vi "main_test3.vi"() -> ()   [LabVIEW 2018]
uses:
  <vilib>/addons/database/Connection.llb/DB Tools Open Connec (Path).vi
  <vilib>/addons/database/NI_Database_API.lvlib
panel:
  in  "确定按钮":bool
  out "数值":dbl format="%#.2g"
  in  "uid":i16
  in  "经度":sgl
  in  "纬度":sgl
  in  "温度":sgl=3.9
  out "时间":timestamp format="%<%H:%M:%S\n%Y/%m/%d>T"
  out "数据采集":bool=TRUE
  out "flaginit":bool=TRUE
  out "温度报警":string[][](table)
  out "疫苗信息":string[][](table)
  out "uid":i16
  out "途径地点":i32
  out "运输路径":cluster{"city":string, "布尔":T1}[](array[cluster])
  out "error out":errorcluster
  out "负责人信息":T2
  in  "CYJ":bool
  out "定位":bool
  out "温度":cluster{"元素":sgl, "温度":sgl, "元素":sgl}(graph)
  out "纬度":string
  out "经度":string
  in  "地图比例":i8(slide)=10 scale=6.0..18.0
  in  "地图":refnum<k7>(container) caption="网页浏览器"
  in  "Setvi":bool
  in  "停止":bool
  # "疫苗冷链储运监控系统\nVACCINE COLD-CHAIN TRANSPORTATION MONITORING SYSTEM"
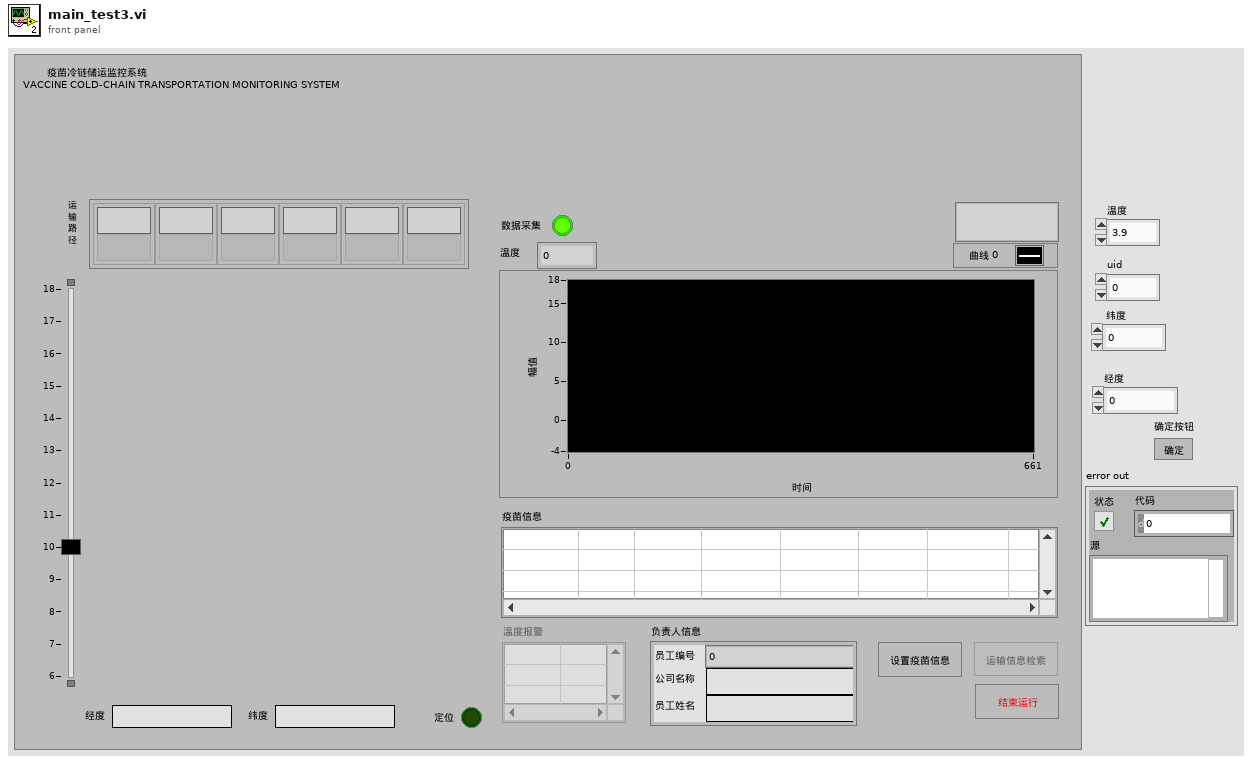
[diagram p1: front panel]
types:
  T1 = typedef "car.ctl" = bool
  T2 = typedef "人员信息.ctl" = cluster{"员工编号":i32, "公司名称":string, "员工姓名":string}
  T3 = typedef "储运信息.ctl" = cluster{"纬度":sgl, "经度":sgl, "温度":sgl, "负责人":i32, "区域":string, "记录时间":timestamp}
  T4 = enum8{"Enabled", "Disabled", "Disabled and Grayed Out"}
  T5 = typedef "NI_Database_API.lvlib/Conn ObjectReference.ctl" = refnum<k1>
  T6 = typedef "疫苗信息.ctl" = cluster{"疫苗名":string, "疫苗编号":i32, "疫苗类型":string, "生产厂家":string, "生产日期":timestamp, "生产地":string, "生产负责人":string, "是否合格":string, "疫苗功能":string}
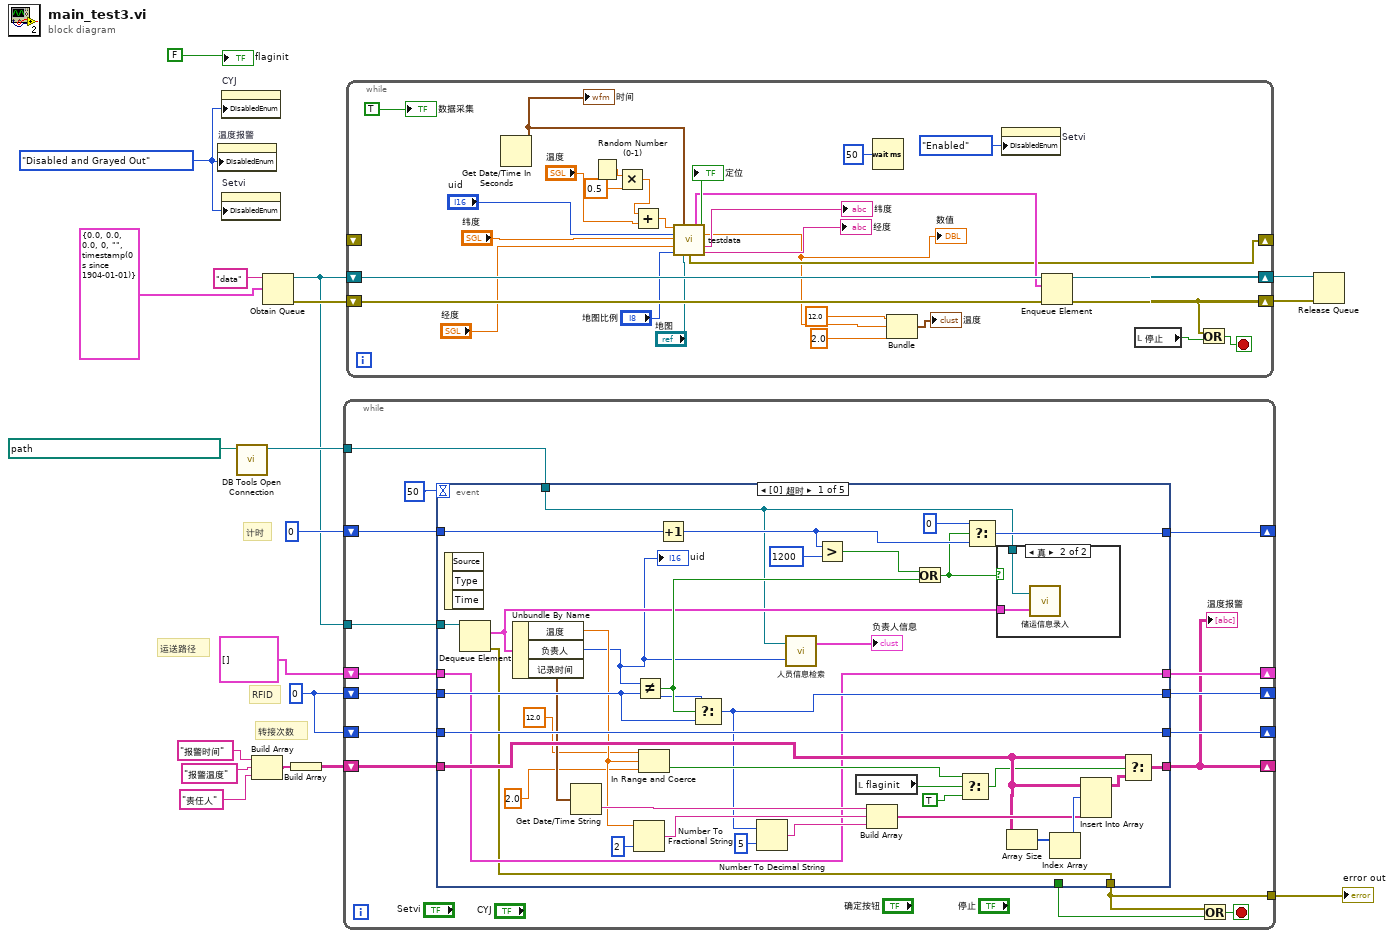
[diagram p0: block diagram]
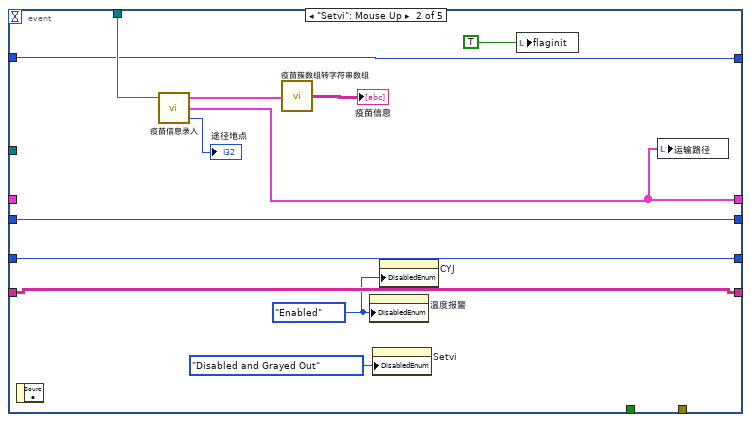
[diagram p3: hidden frame]
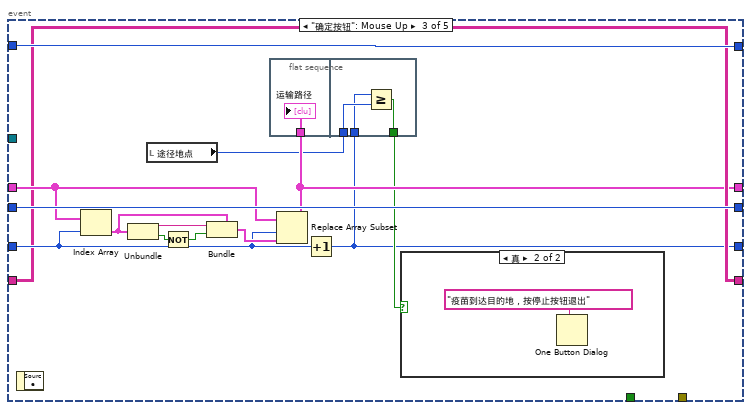
[diagram p4: hidden frame]
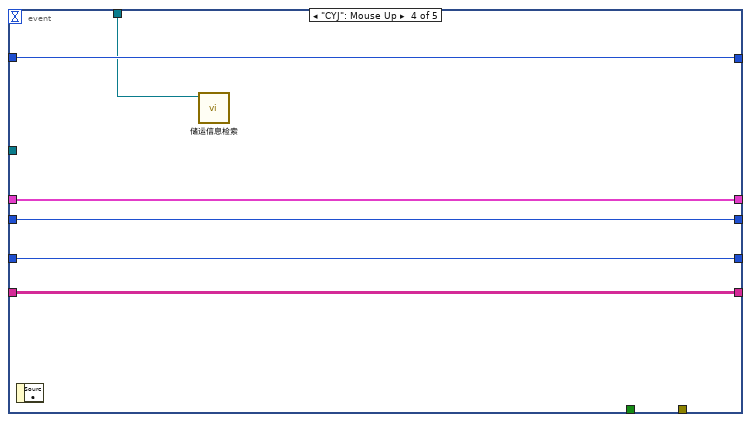
[diagram p6: hidden frame]
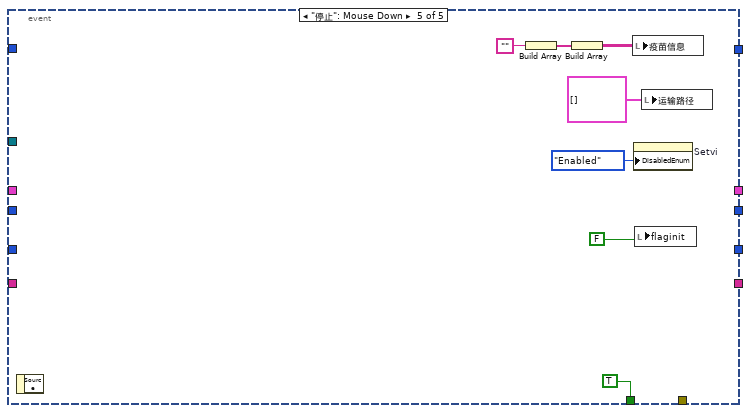
[diagram p7: hidden frame]
diagram:
  w2 = T4."Disabled and Grayed Out" ("禁用")
  w11 = 0
  # "运送路径"
  # "转接次数"
  # "RFID"
  # "计时"
  n1 = property on="温度报警" class="Tbl (严格)"("DisabledEnum"=w2) -> ()  [unwired: 2 in, 2 out]
  n2 = property on="CYJ" class="Bool (严格)"("DisabledEnum"=w2) -> ()  [unwired: 2 in, 2 out]
  n3 = property on="Setvi" class="Bool (严格)"("DisabledEnum"=w2) -> ()  [unwired: 2 in, 2 out]
  n4 = call-poly <vilib>:"DB Tools Open Connection.vi"("connection information"=path "D:/2019毕业设计/Code/GPData.udl" ("路径")) -> ("connection reference"=w14:T5)  [unwired: 7 in, 1 out]
  n5 = Build Array("报警时间", "报警温度", "责任人") -> (w8:string[])
  n6 = Obtain Queue(name (unnamed)="data" ("名称（未命名）"), element data type=T3 {"纬度"=0.0, "经度"=0.0, "温度"=0.0, "负责人"=0, "区域"="", "记录时间"=timestamp(0 s since 1904-01-01)} ("储运信息簇")) -> (queue out=w4:refnum<queue>, error out=w18:errorcluster)  [unwired: 3 in, 1 out]
  n7 = Build Array(w8) -> (w7:string[][])
  n8 = while {
    tunnel: w14 -> [w35]
    shift-right: [w33] -> _
    shift-left: 0 -> [w32]
    shift-right: [w31] -> _
    shift-left: w11 -> [w30]
    tunnel: [w27] -> w12
    shift-right: [w26] -> _
    shift-left: w11 -> [w25]
    shift-right: [w23] -> _
    shift-left: cluster{string, bool}[] [] -> [w24]
    shift-right: [w21] -> _
    shift-left: w7 -> [w22]
    tunnel: w4 -> [w20]
    stop <- w28 stop-if-true
    n9 = event shown="[0] 超时" {
      selector: _ -> [_ _ _ _ _]
      dyn-events: _ -> [_ _ _ _ _]
      timeout: 50 -> [_ _ _ _ _]
      tunnel: w35 -> [w41 w86 _ w106 _]
      tunnel: [_ _ _ _ TRUE] -> w29
      tunnel: [w69 w85 w100 w111 _] -> w33
      tunnel: w32 -> [w72 w85 w100 w111 _]
      tunnel: [w45 w84 w99 w109 _] -> w31
      tunnel: w30 -> [w66 w84 w99 w109 _]
      tunnel: [w38 _ _ _ _] -> w27
      tunnel: [w67 w82 w87 w108 _] -> w26
      tunnel: w25 -> [w67 w82 w92 w108 _]
      tunnel: [w42 w81 w90 w110 _] -> w23
      tunnel: w24 -> [w42 _ w94 w110 _]
      tunnel: w22 -> [w55 w78 w91 w107 _]
      tunnel: [w62 w78 w91 w107 _] -> w21
      tunnel: w20 -> [w49 _ _ _ _]
      event Timeout {
        n10 = event-data() -> ()  [unwired: 1 in, 3 out]
        n11 = Dequeue Element(queue=w49) -> (element=w48:T3, error out=w38:errorcluster)  [unwired: 2 in, 2 out]
        n12 = Unbundle By Name(w48) -> ("温度"=w47:sgl, "负责人"=w40:i32, "记录时间"=w46:timestamp)
        "uid" <- w40
        n13 = Get Date/Time String(seconds (now)=w46) -> (time string=w50:string)  [unwired: 2 in, 1 out]
        n14 = Number To Fractional String(number=w47, precision (6)=i16 2 ("精度(6)")) -> (F-format string=w58:string)  [unwired: 2 in]
        n15 = Not Equal?(x=w40, y=w66) -> (x != y?=w64:bool)
        n16 = In Range and Coerce(upper limit=sgl 12.0 ("上限"), x=w47, lower limit=sgl 2.0 ("下限")) -> (In Range?=w53:bool)  [unwired: 1 out]
        n17 = Increment(x=w72) -> (x+1=w70:i32)
        n18 = Select(t=w40, s=w64, f=w66) -> (s? t:f=w45:i32)
        n19 = Number To Decimal String(number=w45, width (-)=i16 5 ("宽度(-)")) -> (decimal integer string=w44:string)
        n20 = call "人员信息检索.vi"("工作人员编号"=w40, "connection reference"=w41) -> ("负责人数据"=→"负责人信息":T2)  [unwired: 1 out]
        n21 = Greater?(x=w70, y=1200) -> (0:w65:bool)
        n22 = local read "flaginit"() -> (w54:bool)
        n23 = Build Array(w50, w58, w44) -> (w57:string[])
        n24 = Or(x=w65, y=w64) -> (x .or. y?=w63:bool)
        n25 = Select(t=w53, s=w54, f=TRUE) -> (s? t:f=w51:bool)
        n26 = Select(t=0, s=w63, f=w70) -> (s? t:f=w69:i32)
        n27 = case shown="真" w63 {
          tunnel: w41 -> [_ w74]
          tunnel: w48 -> [_ w73]
          frame False {
          }
          frame True {
            n28 = call "储运信息录入.vi"("簇"=w73, "connection reference"=w74) -> ()  [unwired: 1 out]
          }
        }
        n29 = Array Size(array=w55) -> (size(s)=w61:i32[])
        n30 = Index Array(array=w61) -> (element=w60:i32)  [unwired: 1 in]
        n31 = Insert Into Array(array=w55, index (row)=w60, new element=w57) -> (w56:string[][])  [unwired: 1 in]
        n32 = Select(t=w55, s=w51, f=w56) -> (s? t:f=w62:string[][])
      }
      event "Setvi": Mouse Up {
        w75 = T4."Enabled" ("禁用")
        n33 = event-data() -> ()  [unwired: 1 in, 1 out]
        n34 = call "疫苗信息录入.vi"("connection"=w86) -> ("途径地点"=→"途径地点":i32, "运输路线"=w81:cluster{"城市":string, bool}[], "疫苗信息"=w80:T6[])  [unwired: 2 in]
        n35 = call "疫苗簇数组转字符串数组.vi"("疫苗信息"=w80) -> ("疫苗信息"=→"疫苗信息":string[][])
        n36 = property on="温度报警" class="Tbl (严格)"("DisabledEnum"=w75) -> ()  [unwired: 2 in, 2 out]
        n37 = property on="Setvi" class="Bool (严格)"("DisabledEnum"=T4."Disabled and Grayed Out" ("禁用")) -> ()  [unwired: 2 in, 2 out]
        n38 = property on="CYJ" class="Bool (严格)"("DisabledEnum"=w75) -> ()  [unwired: 2 in, 2 out]
        n39 = local write "flaginit"(TRUE) -> ()
        n40 = local write "运输路径"(w81) -> ()
      }
      event "确定按钮": Mouse Up {
        n41 = event-data() -> ()  [unwired: 1 in, 1 out]
        n42 = Index Array(array=w94, index=w92) -> (element=w95:cluster{string, bool})
        n43 = Unbundle(w95) -> (w96:string, w98:bool)
        n44 = local read "途径地点"() -> (w89:i32)
        n45 = Not(x=w98) -> (.not. x?=w97:bool)
        n46 = Bundle(cluster=w95, w96, w97) -> (w93:cluster{string, bool})
        n47 = flat-sequence {
          tunnel: w90 -> [w101]
          tunnel: w89 -> [w104]
          tunnel: [w103] -> w88
          tunnel: w87 -> [w102]
          frame #0 {
            "运输路径" <- w101
          }
          frame #1 {
            n48 = Greater Or Equal?(x=w102, y=w104) -> (x >= y?=w103:bool)
          }
        }
        n49 = Replace Array Subset(array=w94, new element=w93, index=w92) -> (w90:cluster{string, bool}[])
        n50 = Increment(x=w92) -> (x+1=w87:i32)
        n51 = case shown="真" w88 {
          frame False {
          }
          frame True {
            n52 = One Button Dialog(message="疫苗到达目的地，按停止按钮退出" ("消息")) -> ()  [unwired: 1 in, 1 out]
          }
        }
      }
      event "CYJ": Mouse Up {
        n53 = event-data() -> ()  [unwired: 1 in, 1 out]
        n54 = call "储运信息检索.vi"("connection reference"=w106) -> ()  [unwired: 3 in, 3 out]
      }
      event "停止": Mouse Down {
        n55 = event-data() -> ()  [unwired: 1 in, 1 out]
        n56 = Build Array("") -> (w112:string[])
        n57 = Build Array(w112) -> (w113:string[][])
        n58 = local write "疫苗信息"(w113) -> ()
        n59 = property on="Setvi" class="Bool (严格)"("DisabledEnum"=T4."Enabled" ("禁用")) -> ()  [unwired: 2 in, 2 out]
        n60 = local write "flaginit"(FALSE) -> ()
        n61 = local write "运输路径"(cluster{string, bool}[] []) -> ()
      }
    }
    "温度报警" <- w21
    n62 = Or(x=w27, y=w29) -> (x .or. y?=w28:bool)
  }
  "error out" <- w12
  n63 = while {
    shift-right: [w145] -> w17
    shift-left: w4 -> [w147]
    shift-right: [w142] -> w16
    shift-left: w18 -> [w146]
    shift-right: [w128] -> _
    shift-left: _ -> [_]
    stop <- w143 stop-if-true
    n64 = Get Date/Time In Seconds() -> (seconds since 1Jan1904=w132:timestamp)
    "时间" <- w132
    n65 = Random Number (0-1)() -> (number: 0 to 1=w121:dbl)
    n66 = Multiply(x=w121, y=0.5) -> (x*y=w120:dbl)
    n67 = Add(x=w120, y="温度") -> (x+y=w123:dbl)
    n68 = call "testdata.vi"("温度"=w123, "时间"=w132, "uid"="uid", "纬度"="纬度", "经度"="经度", "滑动杆"="地图比例", "地图"="地图") -> ("储运信息簇"=w138:T3, "定位"=→"定位":bool, "温度"=w124:sgl, "纬度显示"=→"纬度":string, "错误输出"=w128:errorcluster, "经度显示"=→"经度":string)  [unwired: 2 in, 1 out]
    "数值" <- w124
    n69 = Wait (ms)(milliseconds to wait=u32 50 ("等待时间（毫秒）")) -> ()  [unwired: 1 out]
    n70 = Bundle("元素"=sgl 12.0, "温度"=w124, "元素"=sgl 2.0) -> (→"温度":cluster{"元素":sgl, "温度":sgl, "元素":sgl})  [unwired: 1 in]
    n71 = property on="Setvi" class="Bool (严格)"("DisabledEnum"=T4."Enabled" ("禁用")) -> ()  [unwired: 2 in, 2 out]
    n72 = Enqueue Element(queue=w147, element=w138, error in (no error)=w146) -> (queue out=w145:refnum<queue>, error out=w142:errorcluster)  [unwired: 1 in, 1 out]
    n73 = local read "停止"() -> (w144:bool)
    n74 = Or(x=w142, y=w144) -> (x .or. y?=w143:bool)
    "数据采集" <- TRUE
  }
  n75 = Release Queue(queue=w17, error in (no error)=w16) -> ()  [unwired: 1 in, 3 out]
  "flaginit" <- FALSE
